vi "Get Auton Files.vi"() -> (3 "All Files in Dir":path[](array[path]))   [LabVIEW 2017]
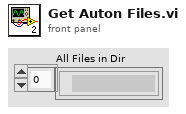
[diagram p1: front panel]
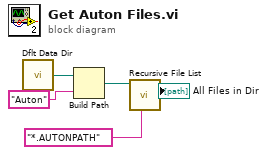
[diagram p0: block diagram]
diagram:
  n1 = call <vilib>:"Dflt Data Dir.vi"() -> ("App:Default Data Directory"=w1:path)
  n2 = Build Path(base path=w1, name or relative path="Auton") -> (appended path=w3:path)
  n3 = call <vilib>:"Recursive File List.vi"("pattern"="*.AUTONPATH", "Folder Path"=w3) -> ("All Files in Dir"=→"All Files in Dir":path[])  [unwired: 5 in, 4 out]
